vi "Report_A131258.vi"(6 "文件重命名":bool, 7 "文件名称":string, 8 "错误输入（无错误）":errorcluster, 10 "合格状态":bool, 11 "布尔数组":bool[][](array[boolean])=[[TRUE]]) -> (0 "error out":errorcluster caption="错误输出")   [LabVIEW 2020]
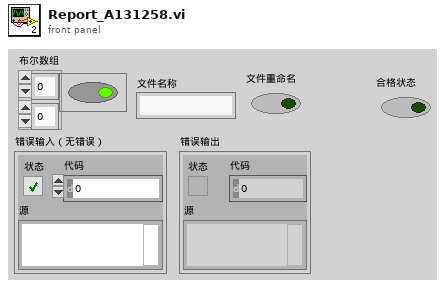
[diagram p1: front panel]
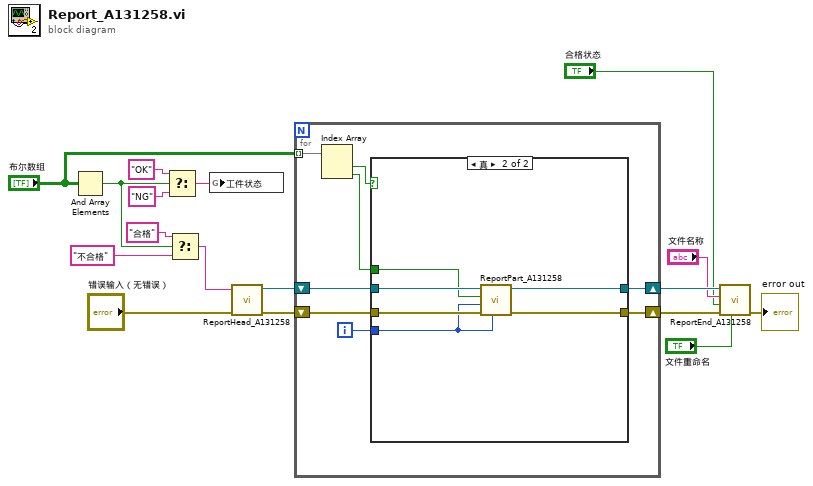
[diagram p0: block diagram]
diagram:
  n1 = And Array Elements(Boolean array="布尔数组") -> (logical AND=w3:bool)
  n2 = Select(t="OK", s=w3, f="NG") -> (s? t:f=w2:string)
  n3 = Select(t="合格", s=w3, f="不合格") -> (s? t:f=w6:string)
  n4 = global write "追溯全部变量.vi" "工件状态"(w2) -> ()
  n5 = call "ReportHead_A131258.vi"("error in (no error)"="错误输入（无错误）", "产品状态"=w6) -> ("error out"=w16:errorcluster, "report out"=w17:refnum<class "NI_report.lvclass">)  [unwired: 8 in]
  n6 = for {
    shift-right: [w23] -> w15
    shift-left: w17 -> [w25]
    shift-right: [w22] -> w14
    shift-left: w16 -> [w24]
    tunnel: "布尔数组" -> [w20] mode=indexing
    i -> [w21]
    n7 = Index Array(array=w20) -> (element #1=w19:bool, element #2=w18:bool)  [unwired: 2 in]
    n8 = case shown="真" w19 {
      tunnel: w25 -> [w26 w33]
      tunnel: w24 -> [w27 w32]
      tunnel: [w26 w31] -> w23
      tunnel: [w27 w30] -> w22
      tunnel: w21 -> [_ w28]
      tunnel: w18 -> [_ w29]
      frame False {
      }
      frame True {
        n9 = call "ReportPart_A131258.vi"("试验项目"=w28, "error in"=w32, "索引"=w28, "合格"=w29, "report in"=w33) -> ("error out 2"=w30:errorcluster, "report out"=w31:refnum<class "NI_report.lvclass">)  [unwired: 5 in]
      }
    }
  }
  n10 = call "ReportEnd_A131258.vi"("文件重命名"="文件重命名", "error in (no error)"=w14, "合格状态"="合格状态", "文件名称"="文件名称", "report in"=w15) -> ("error out"=→"error out":errorcluster)  [unwired: 6 in]
